vi "write_pico_file.vi"(8 "Pico Data In":dbl[][][](array[numeric]), 9 "Raw Data Folder":path, 10 "Filename":string, 11 "Use Channel":bool) -> ()   [LabVIEW 2016]
uses:
  <vilib>/Utility/file.llb/Write Delimited Spreadsheet (DBL).vi
  <vilib>/Utility/file.llb/Write To Spreadsheet File (DBL).vi
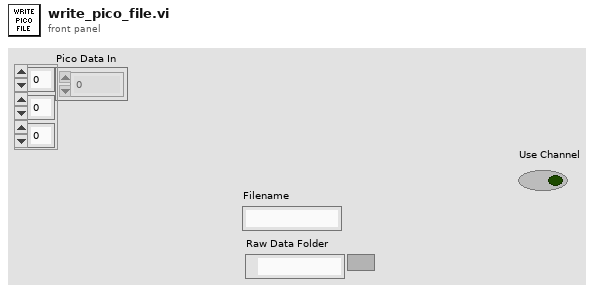
[diagram p1: front panel]
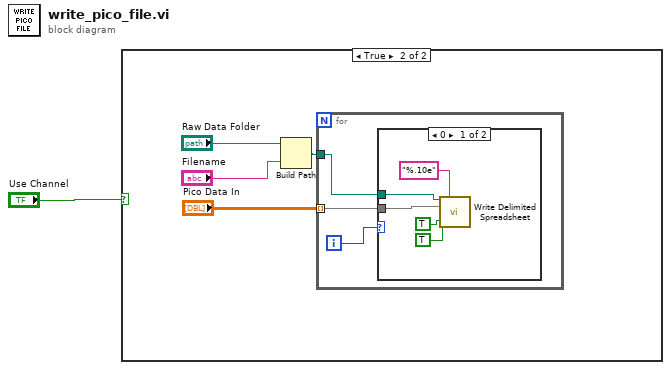
[diagram p0: block diagram]
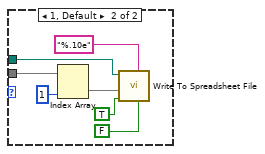
[diagram p3: hidden frame]
diagram:
  n1 = case shown="True" "Use Channel" {
    frame False {
    }
    frame True {
      n2 = Build Path(base path="Raw Data Folder", name or relative path="Filename") -> (appended path=w2:path)
      n3 = for {
        tunnel: "Pico Data In" -> [w7] mode=indexing
        tunnel: w2 -> [w6]
        i -> [w8]
        n4 = case shown="0" w8 {
          tunnel: w7 -> [w13 w18]
          tunnel: w6 -> [w10 w16]
          frame 0 {
            n5 = call-poly <vilib>:"Write Delimited Spreadsheet.vi"("file path (dialog if empty)"=w10, "format (%.3f)"="%.10e", "2D data"=w13, "append to file? (new file:F)"=TRUE ("transpose? (no:F)"), "transpose? (no:F)"=TRUE ("append to file? (new file:F)")) -> ()  [unwired: 9 in, 2 out]
          }
          frame 1, Default {
            n6 = Index Array(array=w18, index (col)=1 ("index (row)")) -> (element=w17:dbl[])  [unwired: 1 in]
            n7 = call-poly <vilib>:"Write To Spreadsheet File.vi"("transpose? (no:F)"=FALSE, "format (%.3f)"="%.10e", "append to file? (new file:F)"=TRUE, "1D data"=w17, "file path (dialog if empty)"=w16) -> ()  [unwired: 3 in, 1 out]
          }
        }
      }
    }
  }
